vi "Display Settings.vi"(11 "ConfigurationThisComponent in":refnum<class "Settings.lvclass">) -> (3 "ConfigurationThisComponent out":refnum<class "Settings.lvclass">)   [LabVIEW 2015, in "Settings.lvclass"]
uses:
  Settings.lvclass
  Typedefs/Serial Settings.ctl
  <userlib>/Common/ILC/Configuration/ADC.ctl
  <userlib>/Common/ILC/Typedefs/ADC Settings.ctl
  <userlib>/Common/ILC/Configuration/Input Channels.ctl
  <userlib>/Common/ILC/Configuration/Scan Rates.ctl
  <userlib>/Common/ILC/Typedefs/DAC Settings.ctl
  Typedefs/PID Settings.ctl
  Typedefs/Closed Loop Settings.ctl
  Typedefs/Pressure Servo Valve Settings.ctl
  Typedefs/Turbo Valve Settings.ctl
  Typedefs/Connection Settings.ctl
  <userlib>/Common/SerialProtocols/Configuration/SerialProtocol.ctl
  <userlib>/Common/Log/Config/Log.ctl
  Typedefs/Hardware Settings.ctl
  Typedefs/Actuator Types.ctl
  Typedefs/Cylinder Types.ctl
  Typedefs/Force Sensor Settings.ctl
  <userlib>/Common/Devices/ForceSensorCalculator/Config/ForceSensorCalculator.ctl
  <userlib>/Common/ILC/Configuration/ILCConfiguration.lvlib
  <userlib>/Common/ILC/Typedefs/ILCTypedefs.lvlib
  Typedefs/FAMT Typedefs.lvlib
  <userlib>/Common/SerialProtocols/SerialProtocols.lvlib
  <userlib>/Common/Log/Log.lvlib
  <userlib>/Common/Devices/ForceSensorCalculator/ForceSensorCalculator.lvlib
panel:
  in  "ctrlRefArrayUsrEvnt":refnum<user-event>
  in  "ConfigTab":T1(tab)
  in  "TestDataLog":T2={"Log Directory"=path "", "Log Filename Base"="", "Max records per file"=1000, "Comment"=""} {"Max records per file" min=100 max=1000000}
  in  "ILC Serial Settings":T3={"Baud Rate"=9600, "Data Bits"=8, "Parity"=enum."None", "Flow Control"=0, "Stop Bits"=10, "Timeout (ms)"=10000, "Byte Count"=200, "Enable Termination Character"=FALSE, "Termination Char"=200} {"Termination Char" format="%x"; "Stop Bits" items=["1.0"=10, "1.5"=15, "2.0"=20]; "Flow Control" items=["None", "XON/XOFF", "RTS/CTS", "XON/XOFF & RTS/CTS", "DTR/DSR", "XON/XOFF & DTR/DSR"]; "Data Bits" min=5 max=8 step=1}
  in  "Tovey Serial Settings":T3={"Baud Rate"=9600, "Data Bits"=8, "Parity"=enum."None", "Flow Control"=0, "Stop Bits"=10, "Timeout (ms)"=10000, "Byte Count"=200, "Enable Termination Character"=FALSE, "Termination Char"=200} caption="TEI9150" {"Termination Char" format="%x"; "Stop Bits" items=["1.0"=10, "1.5"=15, "2.0"=20]; "Flow Control" items=["None", "XON/XOFF", "RTS/CTS", "XON/XOFF & RTS/CTS", "DTR/DSR", "XON/XOFF & DTR/DSR"]; "Data Bits" min=5 max=8 step=1}
  in  "ILC ADC Settings":T4={"Reference Voltage Vref"=0.0, "Nominal Input Range in Counts"=128, "Preamplifier Gain"=0, "Conversion Settling Cycles"=0} {"Conversion Settling Cycles" min=1; "Preamplifier Gain" min=1; "Nominal Input Range in Counts" min=128; "Reference Voltage Vref" min=-10.0 max=10.0 format="%.3f"}
  in  "ILC DAC Settings":T5={"Voltage Reference"=4.096, "Min Counts"=0, "Max Counts"=65535} {"Voltage Reference" format="%.3f"}
  in  "ILC Default Settings":T6 {"PGA Gain Coefficient" max=7}
  in  "Pressure Servo Settings":T9={"Center Point"=2.5, "Area"=0.004536, "PA to PSI"=0.000145038, "Off Value"=0.004536} {"Off Value" format="%.3f"; "PA to PSI" format="%.9f"; "Area" format="%.9f"; "Center Point" format="%.3f"}
  in  "Turbo Valve Settings":T10={"Bias"=70, "Minimum Voltage"=0.0, "Maximum Voltage"=4.096, "Off Value"=0.0} {"Off Value" format="%.3f"; "Maximum Voltage" format="%.3f"; "Minimum Voltage" format="%.3f"; "Bias" step=1}
  in  "PID Settings":T11={"Pressure Servo Valve Settings"={"P"=1.0, "I"=0.1, "D"=0.0, "Minimum"=0.0, "Maximum"=10.0}, "Turbo Valve Settings"={"P"=1.0, "I"=0.1, "D"=0.0, "Minimum"=0.0, "Maximum"=10.0}} {"Turbo Valve Settings"."Maximum" format="%.6f"; "Turbo Valve Settings"."Minimum" format="%.6f"; "Turbo Valve Settings"."D" format="%.6f"; "Turbo Valve Settings"."I" format="%.6f"; "Turbo Valve Settings"."P" format="%.6f"; "Pressure Servo Valve Settings"."Maximum" format="%.6f"; "Pressure Servo Valve Settings"."Minimum" format="%.6f"; "Pressure Servo Valve Settings"."D" format="%.6f"; "Pressure Servo Valve Settings"."I" format="%.6f"; "Pressure Servo Valve Settings"."P" format="%.6f"}
  in  "Force Sensor Settings":T13={"Reference Voltage Vref"=0.0, "FC1 Force Sensor"={"Capacity"=1.0, "Sensitivity"=0.001}, "FC2 Force Sensor"={"Capacity"=1.0, "Sensitivity"=0.001}} {"FC2 Force Sensor"."Sensitivity" min=0.001 max=5000.0 format="%.4f"; "FC2 Force Sensor"."Capacity" min=1.0 max=5000000.0 format="%.4f"; "FC1 Force Sensor"."Sensitivity" min=0.001 max=5000.0 format="%.4f"; "FC1 Force Sensor"."Capacity" min=1.0 max=5000000.0 format="%.4f"; "Reference Voltage Vref" min=-10.0 max=10.0 format="%.3f"}
  in  "Connection Settings":T15={"Pressure Servo Valve 1 DAC"=1, "Pressure Servo Valve 2 DAC"=2, "Turbo Valve DAC"=3, "Load Cell ADC"=2, "FC1 ILC Port"="", "FC2 ILC Port"="", "Tovey A-B Port"="", "Tovey C-F Port"="", "Tovey D-E Port"="", "FC1 ILC Protocol"=enum."RS485", "FC2 ILC Protocol"=enum."RS485", "Tovey A-B Protocol"=enum."RS485", "Tovey C-F Protocol"=enum."RS485", "Tovey D-E Protocol"=enum."RS485", "Tovey A-B Address"=3, "Tovey C-F Address"=1, "Tovey D-E Address"=1, "Bias DAC"=4} {"Bias DAC" min=1 max=4; "Tovey D-E Address" min=1; "Tovey C-F Address" min=1; "Tovey A-B Address" min=1; "Load Cell ADC" min=1 max=4; "Turbo Valve DAC" min=1 max=4; "Pressure Servo Valve 2 DAC" min=1 max=4; "Pressure Servo Valve 1 DAC" min=1 max=4}
  in  "Hardware Settings":T17
  # "Gain is 2^gain_coefficient"
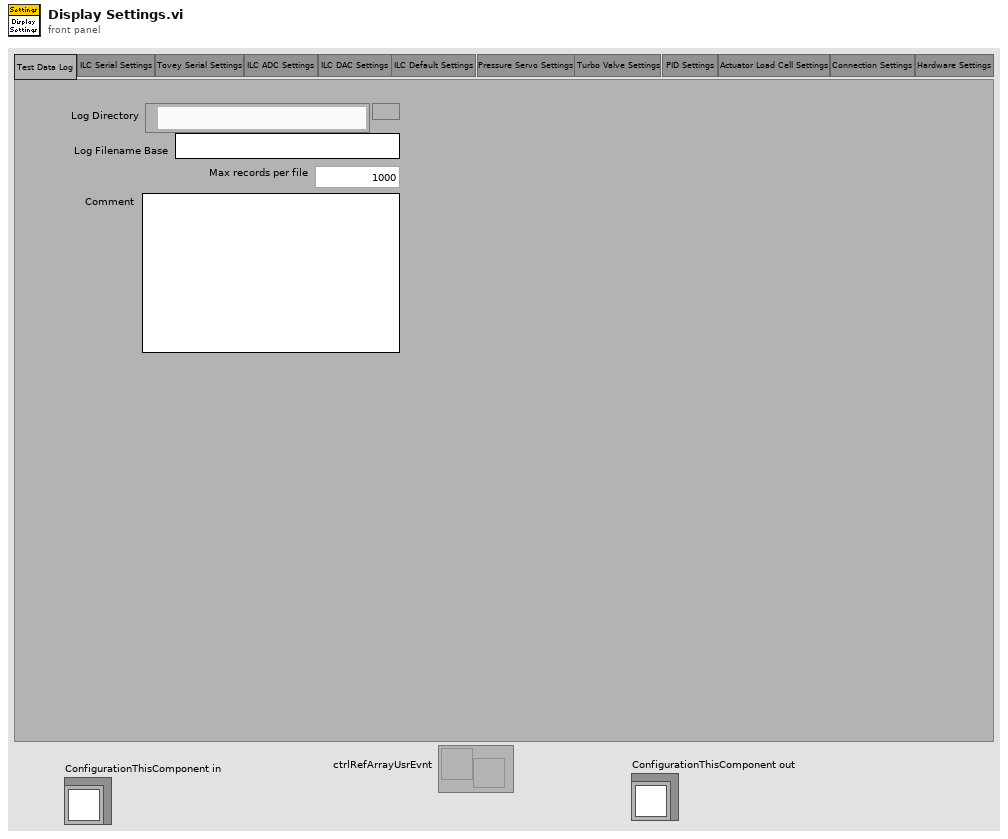
[diagram p1: front panel]
types:
  T1 = enum32{"Test Data Log", "ILC Serial Settings", "Tovey Serial Settings", "ILC ADC Settings", "ILC DAC Settings", "ILC Default Settings", "Pressure Servo Settings", "Turbo Valve Settings", "PID Settings", "Actuator Load Cell Settings", "Connection Settings", "Hardware Settings"}
  T2 = typedef "Log.lvlib/Log.ctl" = cluster{"Log Directory":path, "Log Filename Base":string, "Max records per file":u32, "Comment":string}
  T3 = typedef "FAMT Typedefs.lvlib/Serial Settings.ctl" = cluster{"Baud Rate":u32, "Data Bits":u16, "Parity":enum16{"None", "Odd", "Even", "Mark", "Space"}, "Flow Control":u16, "Stop Bits":u16, "Timeout (ms)":u32, "Byte Count":u32, "Enable Termination Character":bool, "Termination Char":u8}
  T4 = typedef "ILCCommon.lvlib/ILCConfiguration.lvlib/ADC.ctl" = cluster{"Reference Voltage Vref":dbl[unit], "Nominal Input Range in Counts":u32, "Preamplifier Gain":u8, "Conversion Settling Cycles":u16}
  T5 = typedef "ILCCommon.lvlib/ILCTypedefs.lvlib/DAC Settings.ctl" = cluster{"Voltage Reference":dbl[unit], "Min Counts":i32, "Max Counts":i32}
  T6 = typedef "ILCCommon.lvlib/ILCTypedefs.lvlib/ADC Settings.ctl" = cluster{"Input Channels":T7, "Scan Rate (Hz) ":T8, "PGA Gain Coefficient":u8}
  T7 = typedef "ILCCommon.lvlib/ILCConfiguration.lvlib/Input Channels.ctl" = enum16{"Channel 0", "3 Channels", "5 Channels"}
  T8 = typedef "ILCCommon.lvlib/ILCConfiguration.lvlib/Scan Rates.ctl" = enum16{"50", "60", "100", "120", "200", "240", "300", "400", "480", "600", "1200", "2400", "4800"}
  T9 = typedef "FAMT Typedefs.lvlib/Pressure Servo Valve Settings.ctl" = cluster{"Center Point":dbl[unit], "Area":dbl, "PA to PSI":dbl, "Off Value":dbl}
  T10 = typedef "FAMT Typedefs.lvlib/Turbo Valve Settings.ctl" = cluster{"Bias":u16, "Minimum Voltage":dbl, "Maximum Voltage":dbl, "Off Value":dbl}
  T11 = typedef "FAMT Typedefs.lvlib/PID Settings.ctl" = cluster{"Pressure Servo Valve Settings":T12, "Turbo Valve Settings":T12}
  T12 = typedef "FAMT Typedefs.lvlib/Closed Loop Settings.ctl" = cluster{"P":dbl, "I":dbl, "D":dbl, "Minimum":dbl, "Maximum":dbl}
  T13 = typedef "FAMT Typedefs.lvlib/Force Sensor Settings.ctl" = cluster{"Reference Voltage Vref":dbl[unit], "FC1 Force Sensor":T14, "FC2 Force Sensor":T14}
  T14 = typedef "ForceSensorCalculator.lvlib/ForceSensorCalculator.ctl" = cluster{"Capacity":dbl[unit], "Sensitivity":dbl[unit]}
  T15 = typedef "FAMT Typedefs.lvlib/Connection Settings.ctl" = cluster{"Pressure Servo Valve 1 DAC":u8, "Pressure Servo Valve 2 DAC":u8, "Turbo Valve DAC":u8, "Load Cell ADC":u8, "FC1 ILC Port":refnum<visa-resource-name>, "FC2 ILC Port":refnum<visa-resource-name>, "Tovey A-B Port":refnum<visa-resource-name>, "Tovey C-F Port":refnum<visa-resource-name>, "Tovey D-E Port":refnum<visa-resource-name>, "FC1 ILC Protocol":T16, "FC2 ILC Protocol":T16, "Tovey A-B Protocol":T16, "Tovey C-F Protocol":T16, "Tovey D-E Protocol":T16, "Tovey A-B Address":u8, "Tovey C-F Address":u8, "Tovey D-E Address":u8, "Bias DAC":u8}
  T16 = typedef "SerialProtocols.lvlib/SerialProtocol.ctl" = enum16{"RS232", "RS485", "SerialSimulator"}
  T17 = typedef "FAMT Typedefs.lvlib/Hardware Settings.ctl" = cluster{"Actuator Types":T18, "Cylinder Types":T19, "Calibrated Load Cell Moment":dbl[unit]}
  T18 = typedef "FAMT Typedefs.lvlib/Actuator Types.ctl" = enum16{"Single", "Dual"}
  T19 = typedef "FAMT Typedefs.lvlib/Cylinder Types.ctl" = enum16{"PSV Open", "PSV Closed", "TV Open", "TV Closed", "Closed"}
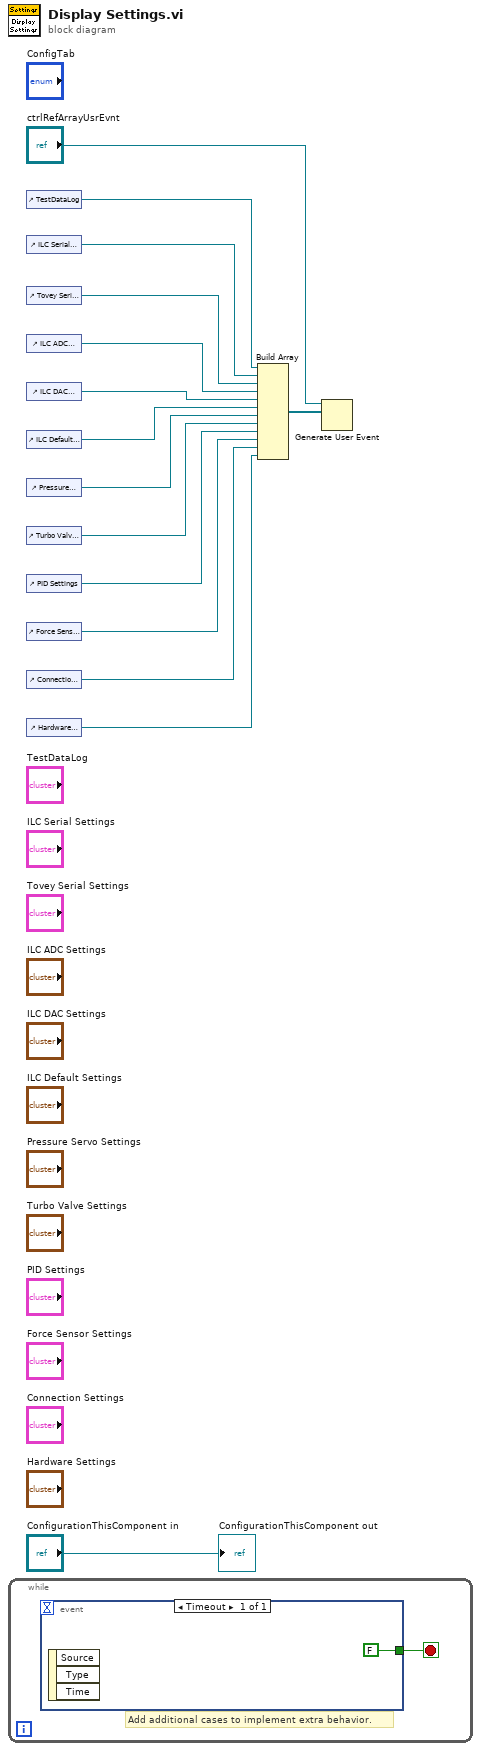
[diagram p0: block diagram]
diagram:
  n1 = while {
    stop <- w16 stop-if-true
    # "Add additional cases to implement extra behavior."
    n2 = event shown="[0] Timeout" {
      selector: _ -> [_]
      dyn-events: _ -> [_]
      timeout: _ -> [_]
      tunnel: [FALSE] -> w16
      event Timeout {
        n3 = event-data() -> ()  [unwired: 1 in, 3 out]
      }
    }
  }
  n4 = control-ref of="TestDataLog"() -> (w5:refnum<vi>)
  n5 = control-ref of="ILC Serial Settings"() -> (w6:refnum<vi>)
  n6 = control-ref of="Tovey Serial Settings"() -> (w7:refnum<vi>)
  n7 = control-ref of="ILC ADC Settings"() -> (w13:refnum<vi>)
  n8 = control-ref of="ILC DAC Settings"() -> (w4:refnum<vi>)
  n9 = control-ref of="ILC Default Settings"() -> (w12:refnum<vi>)
  n10 = control-ref of="Pressure Servo Settings"() -> (w10:refnum<vi>)
  n11 = control-ref of="Turbo Valve Settings"() -> (w9:refnum<vi>)
  n12 = control-ref of="PID Settings"() -> (w3:refnum<vi>)
  n13 = control-ref of="Force Sensor Settings"() -> (w1:refnum<vi>)
  n14 = control-ref of="Connection Settings"() -> (w8:refnum<vi>)
  n15 = control-ref of="Hardware Settings"() -> (w2:refnum<vi>)
  n16 = Build Array(w5, w6, w7, w13, w4, w12, w10, w9, w3, w1, w8, w2) -> (w11:refnum<vi>[])
  n17 = Generate User Event(user event="ctrlRefArrayUsrEvnt", event data cluster=w11) -> ()  [unwired: 2 in, 2 out]
  "ConfigurationThisComponent out" <- "ConfigurationThisComponent in"
